vi "DataA_B.vi"(8 "error in (no error)":errorcluster, 11 "VISA resource name":refnum<visa-resource-name>) -> (0 "error out":errorcluster, 1 "MKRB":dbl, 2 "MKRA":dbl, 3 "VISA resource name out":refnum<visa-resource-name>)   [LabVIEW 2017]
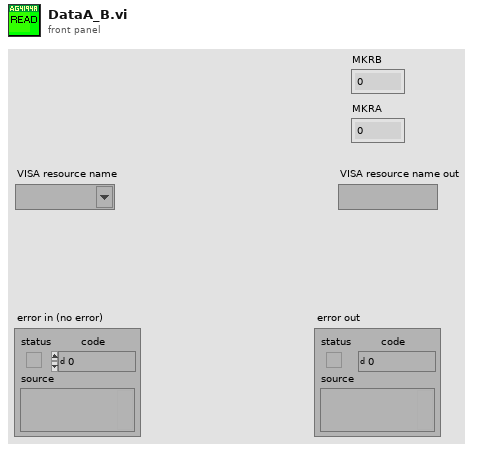
[diagram p1: front panel]
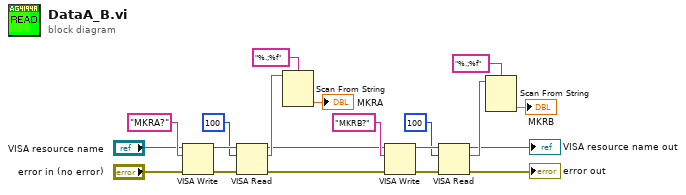
[diagram p0: block diagram]
diagram:
  n1 = VISA Write(VISA resource name="VISA resource name", write buffer="MKRA?" ("write buffer (\"\")"), error in (no error)="error in (no error)") -> (VISA resource name out=w15:refnum<visa-resource-name>, error out=w16:errorcluster)  [unwired: 1 out]
  n2 = VISA Read(VISA resource name=w15, byte count=u32 100 ("byte count (0)"), error in (no error)=w16) -> (VISA resource name out=w8:refnum<visa-resource-name>, read buffer=w12:string, error out=w7:errorcluster)  [unwired: 1 out]
  n3 = Scan From String(format string="%.;%f", input string=w12) -> (output 1=→"MKRA":dbl)  [unwired: 3 in, 3 out]
  n4 = VISA Write(VISA resource name=w8, write buffer="MKRB?" ("write buffer (\"\")"), error in (no error)=w7) -> (VISA resource name out=w19:refnum<visa-resource-name>, error out=w20:errorcluster)  [unwired: 1 out]
  n5 = VISA Read(VISA resource name=w19, byte count=u32 100 ("byte count (0)"), error in (no error)=w20) -> (VISA resource name out=→"VISA resource name out":refnum<visa-resource-name>, read buffer=w9:string, error out=→"error out":errorcluster)  [unwired: 1 out]
  n6 = Scan From String(format string="%.;%f", input string=w9) -> (output 1=→"MKRB":dbl)  [unwired: 3 in, 3 out]
